vi "waitStopServerOcc.vi"(8 "error in (no error)":errorcluster, 11 "TcpServerTel in":refnum<class "TcpServerTel.lvclass">) -> (0 "error out":errorcluster, 2 "stopServer":bool, 3 "TcpServerTel out":refnum<class "TcpServerTel.lvclass">)   [LabVIEW 2018, in "TcpServerTel.lvclass"]
doc: "Wait to stop the runServer.vi. This is a non-block call function."
uses:
  TcpServerTel.lvclass
  home/pcortes/github/ts_labview_tcp_json/src/TcpServerBase/TcpServerBase.lvclass
  TcpServerBase/TcpServerBase.lvclass/TcpServerBase.ctl
  TcpServerBase/TcpServerBase.lvclass
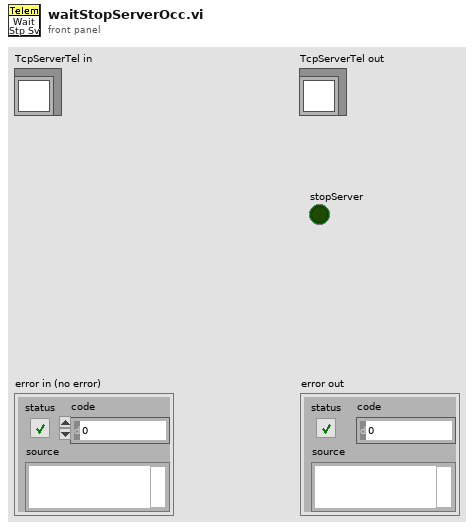
[diagram p1: front panel]
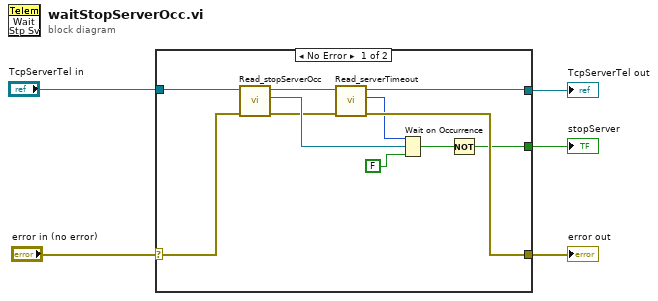
[diagram p0: block diagram]
diagram:
  n1 = case shown="No Error" "error in (no error)" {
    selector: "error in (no error)" -> [w15 w18]
    tunnel: "TcpServerTel in" -> [w16 w17]
    tunnel: [w8 w18] -> w3
    tunnel: [w9 w17] -> w2
    tunnel: [w7 _] -> w1
    frame No Error {
      n2 = call "Read_stopServerOcc.vi"("error in (no error)"=w15, "TcpServerBase in"=w16) -> ("error out"=w10:errorcluster, "stopServerOcc"=w12:refnum<k4>, "TcpServerBase out"=w11:refnum<class "TcpServerTel.lvclass">)  [unwired: 7 in]
      n3 = call "Read_serverTimeout.vi"("error in (no error)"=w10, "TcpServerBase in"=w11) -> ("error out"=w8:errorcluster, "serverTimeout"=w6:i32, "TcpServerBase out"=w9:refnum<class "TcpServerTel.lvclass">)  [unwired: 7 in]
      n4 = Wait on Occurrence(1:FALSE ("ignore previous (T)"), 2:w12, 3:w6) -> (0:w13:bool)
      n5 = Not(x=w13) -> (.not. x?=w7:bool)
    }
    frame Error {
    }
  }
  "error out" <- w3
  "TcpServerTel out" <- w2
  "stopServer" <- w1
